vi "Get Command From String.vi"(11 "String":string) -> (2 "Arguments":variant, 3 "Command":string)   [LabVIEW 2017, in "Message Interface.lvlib" / "Command.lvclass"]
uses:
  Command.lvclass
  Volumes/Data/Users/benji667/Git/BuildFarm/BuildWorker/Classes/iMessage/iMessage.lvclass
  Command.lvclass/Command.ctl
  iMessage/iMessage.lvclass
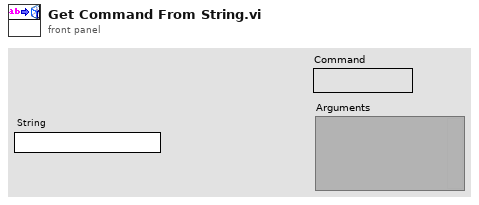
[diagram p1: front panel]
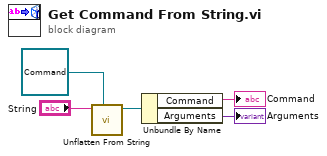
[diagram p0: block diagram]
diagram:
  n1 = call "Unflatten From String.vi"("iMessage in"=refnum<class "Command.lvclass"> refnum ("Command in"), "binary string"="String") -> ("iMessage out"=w3:refnum<class "Command.lvclass">)  [unwired: 8 in, 1 out]
  n2 = Unbundle By Name(w3) -> ("Command"=→"Command":string, "Arguments"=→"Arguments":variant)
